vi "WPI_PWMSafetyError.vi"(0 "PWMDeviceRef":T1={"DeviceStatus"={"status"=FALSE, "code"=0, "source"=""}, "PWM Channel"=enum."PWM 1"}) -> (4 "PWMDeviceRef":T1={"DeviceStatus"={"status"=FALSE, "code"=0, "source"=""}, "PWM Channel"=enum."PWM 1"})   [LabVIEW 2017]
doc: "This subVI does two things:\n1. It builds up output specific information to help locate the problem.\n2. It calls the FRC Build Error, so all the information gets passed to the Driver Station."
uses:
  <vilib>/Rock Robotics/WPI/PWM/WPI_PWMDeviceRef.ctl
  <vilib>/Rock Robotics/SystemInterfaces/DIO/FPGA_DIOPWMChannel.ctl
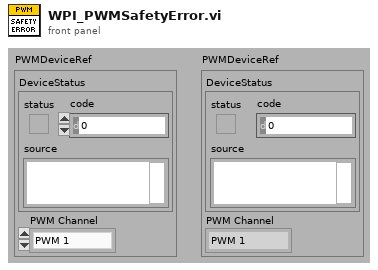
[diagram p1: front panel]
types:
  T1 = typedef "WPI_PWMDeviceRef.ctl" = cluster{"DeviceStatus":errorcluster, "PWM Channel":T2}
  T2 = typedef "FPGA_DIOPWMChannel.ctl" = enum8{"PWM 0", "PWM 1", "PWM 2", "PWM 3", "PWM 4", "PWM 5", "PWM 6", "PWM 7", "PWM 8", "PWM 9", "PWM MXP 0", "PWM MXP 1", "PWM MXP 2", "PWM MXP 3", "PWM MXP 4", "PWM MXP 5", "PWM MXP 6", "PWM MXP 7", "PWM MXP 8", "PWM MXP 9", "Invalid"}
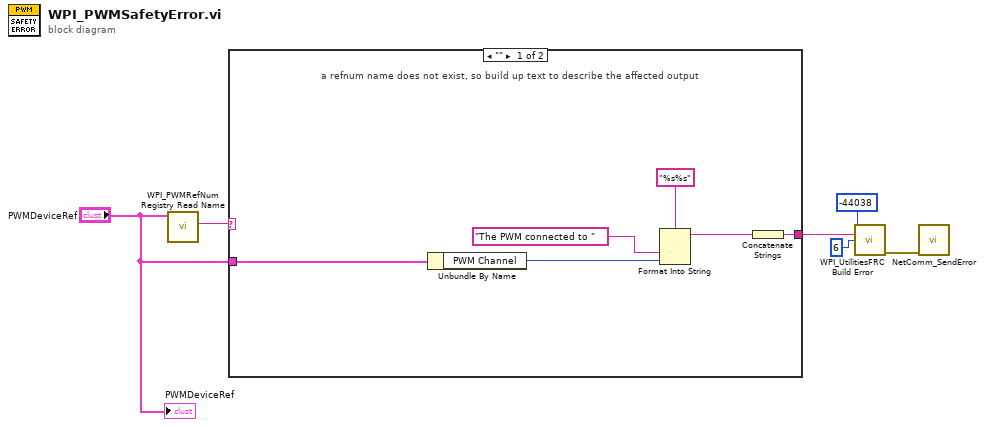
[diagram p0: block diagram]
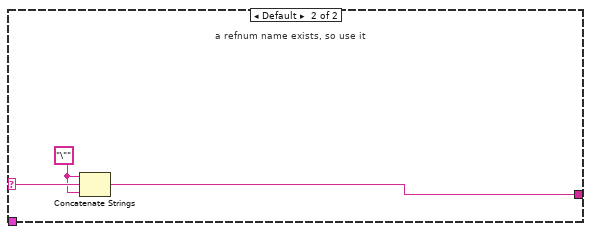
[diagram p2: hidden frame]
diagram:
  n1 = call <vilib>:"WPI_PWMRefNum Registry Read Name.vi"("PWMDeviceRef"="PWMDeviceRef") -> ("refnum name"=w4:string)  [unwired: 1 in, 9 out]
  n2 = case shown="\"\"" w4 {
    selector: w4 -> [_ w15]
    tunnel: [w11 w14] -> w3
    tunnel: "PWMDeviceRef" -> [w10 _]
    frame "" {
      # "a refnum name does not exist, so build up text to describe the affected output"
      n3 = Unbundle By Name(w10) -> ("PWM Channel"=w8:T2)
      n4 = Format Into String(format string="%s%s", "The PWM connected to " ("format string"), w8) -> (resulting string=w12:string)  [unwired: 2 in, 1 out]
      n5 = Concatenate Strings(w12) -> (w11:string)
    }
    frame Default {
      w13 = "\"" ("string")
      # "a refnum name exists, so use it"
      n6 = Concatenate Strings(w13, w15, w13) -> (w14:string)
    }
  }
  n7 = call <vilib>:"WPI_UtilitiesFRC Build Error.vi"("error code"=-44038 ("code"), "extra error text"=w3, "chain levels to remove (1)"=6) -> ("error out"=w1:errorcluster)  [unwired: 3 in, 9 out]
  n8 = call <vilib>:"NetComm_SendError.vi"("error in (no error)"=w1) -> ()  [unwired: 11 in]
  "PWMDeviceRef" <- "PWMDeviceRef"
